vi "Add Contents In Tree.vi"(4 "Symbol Index":i32, 6 "Node Name":string, 8 "error in (no error)":errorcluster, 9 "Node ID":string, 10 "Parent Node":string, 11 "Browers in":refnum<class "Browers Controller.lvclass">) -> (0 "error out":errorcluster, 3 "Browers out":refnum<class "Browers Controller.lvclass">)   [LabVIEW 2015, in "Browers Controller.lvclass"]
uses:
  Browers Controller.lvclass
  Browers Controller.lvclass/Browers Controller.ctl
  Brower View/Brower View.lvclass/Brower View.ctl
  MyTreeAPI/MyTreeAPI.lvclass
  Brower View/Brower View.lvclass
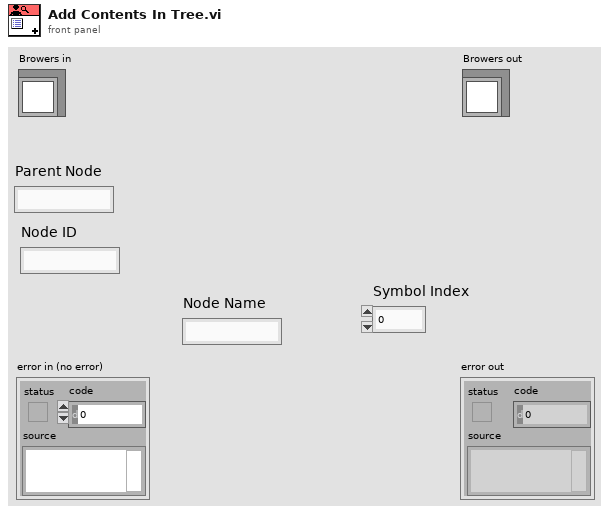
[diagram p1: front panel]
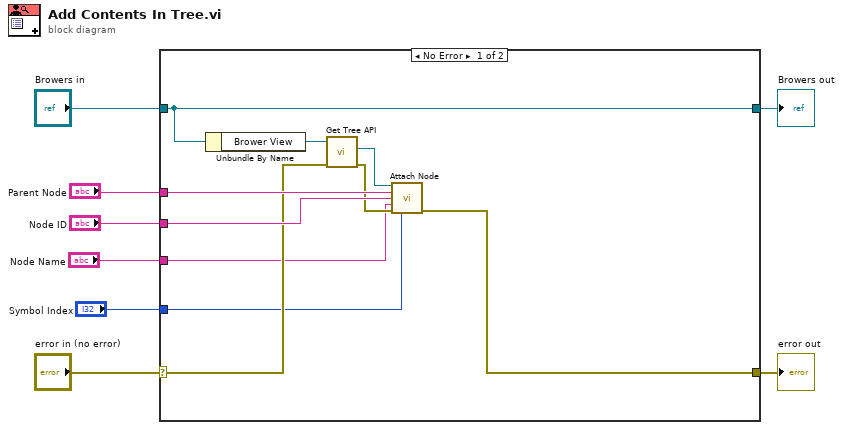
[diagram p0: block diagram]
diagram:
  n1 = case shown="No Error" "error in (no error)" {
    selector: "error in (no error)" -> [w13 w20]
    tunnel: [w11 w20] -> w7
    tunnel: [w14 w19] -> w5
    tunnel: "Browers in" -> [w14 w19]
    tunnel: "Parent Node" -> [w18 _]
    tunnel: "Node ID" -> [w17 _]
    tunnel: "Symbol Index" -> [w9 _]
    tunnel: "Node Name" -> [w10 _]
    frame No Error {
      n2 = Unbundle By Name(w14) -> ("Brower View"=w15:refnum<class "Brower View.lvclass">)
      n3 = call "Get Tree API.vi"("error in (no error)"=w13, "Brower View in"=w15) -> ("error out"=w12:errorcluster, "myTree.lvclass"=w16:refnum<class "MyTreeAPI.lvclass">)  [unwired: 7 in, 1 out]
      n4 = call "Attach Node.vi"("TREE in"=w16, "Parent Node"=w18, "Node ID"=w17, "Node Name"=w10, "error in (no error)"=w12, "Symbol Index"=w9) -> ("error out"=w11:errorcluster)  [unwired: 7 in, 2 out]
    }
    frame Error {
    }
  }
  "error out" <- w7
  "Browers out" <- w5
